vi "DefaultUnwired.vi"() -> ()   [LabVIEW 2021]
panel:
  in  "Numeric":u8
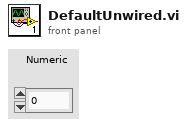
[diagram p1: front panel]
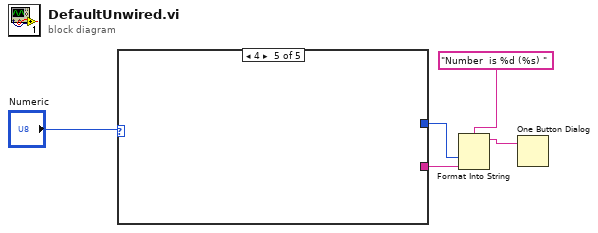
[diagram p0: block diagram]
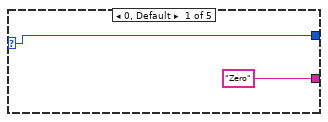
[diagram p2: hidden frame]
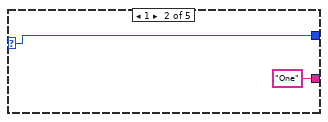
[diagram p3: hidden frame]
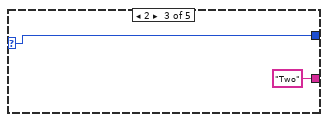
[diagram p4: hidden frame]
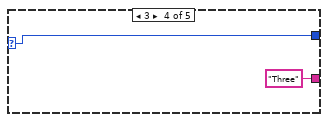
[diagram p5: hidden frame]
diagram:
  n1 = case shown="4" "Numeric" {
    selector: "Numeric" -> [w7 w9 w11 w13 _]
    tunnel: [w7 w9 w11 w13 _] -> w2
    tunnel: ["Zero" "One" "Two" "Three" _] -> w1
    frame 0, Default {
    }
    frame 1 {
    }
    frame 2 {
    }
    frame 3 {
    }
    frame 4 {
    }
  }
  n2 = Format Into String(format string="Number  is %d (%s) ", w2, w1) -> (resulting string=w3:string)  [unwired: 2 in, 1 out]
  n3 = One Button Dialog(message=w3) -> ()  [unwired: 1 in, 1 out]
